vi "Graph Buffer.vi"(4 "Channel Names":string[](array[string]), 5 "Channels":T2, 6 "Data":sgl[](array[numeric]) format="%.2f", 7 "X Range":T3) -> (0 "LastValues":T1, 1 "Graph 2":sgl[][](array[numeric]) format="%.2f", 3 "Graph 1":sgl[][](array[numeric]) format="%.2f")   [LabVIEW 2015]
doc: "This VI acts as a buffer for the Housekeeping data, maintaining a record of the last 120 minutes of data and putting out the requested graphs.\n\nHK Buffer.vi by David Thomson Original Code Consulting\n September 2002 www.originalcode.com"
uses:
  X Range.ctl
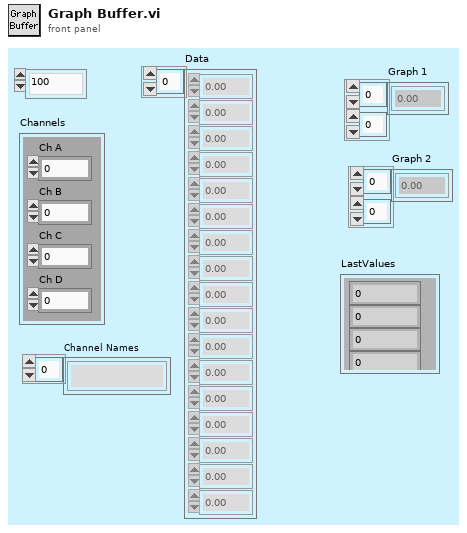
[diagram p1: front panel]
types:
  T1 = cluster{"Ch0":sgl, "Ch1":sgl, "Ch2":sgl, "Ch3":sgl}
  T2 = cluster{"Ch A":i32, "Ch B":i32, "Ch C":i32, "Ch D":i32}
  T3 = typedef "X Range.ctl" = enum16{"100", "300", "500", "1000", "3000", "5000", "10000", "20000", "30000", "40000", "60000"}
  T4 = cluster{"RT Channel":sgl, "RT Channel":sgl, "RT Channel":sgl, "RT Channel":sgl}
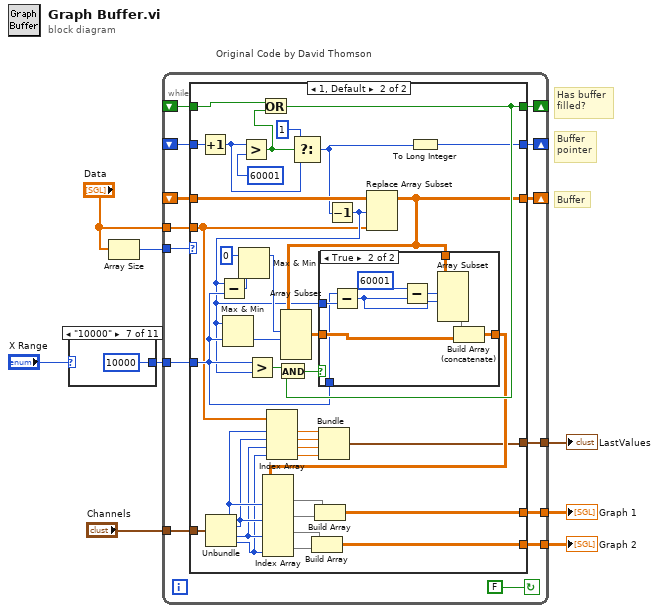
[diagram p0: block diagram]
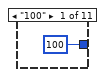
[diagram p2: hidden frame]
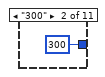
[diagram p3: hidden frame]
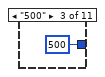
[diagram p4: hidden frame]
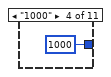
[diagram p5: hidden frame]
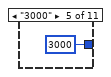
[diagram p6: hidden frame]
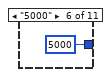
[diagram p7: hidden frame]
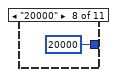
[diagram p8: hidden frame]
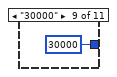
[diagram p9: hidden frame]
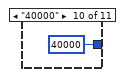
[diagram p10: hidden frame]
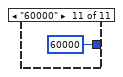
[diagram p11: hidden frame]
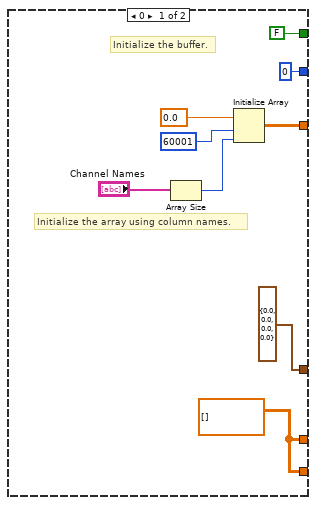
[diagram p12: hidden frame]
diagram:
  # "Buffer"
  # "Buffer\npointer"
  # "Has buffer\nfilled?"
  n1 = case shown="\"10000\"" "X Range" {
    tunnel: [100 ("y") 300 ("y") 500 ("y") 1000 ("y") 3000 ("y") 5000 ("y") 10000 ("y") 20000 ("y") 30000 ("y") 40000 ("y") 60000 ("y")] -> w5
    frame "100" {
    }
    frame "300" {
    }
    frame "500" {
    }
    frame "1000" {
    }
    frame "3000" {
    }
    frame "5000" {
    }
    frame "10000" {
    }
    frame "20000" {
    }
    frame "30000" {
    }
    frame "40000" {
    }
    frame "60000" {
    }
  }
  n2 = Array Size(array="Data") -> (size(s)=w8:i32)
  n3 = while "Original Code by David Thomson" {
    shift-right: [w31] -> _
    shift-left: _ -> [w29]
    shift-right: [w30] -> _
    shift-left: _ -> [w28]
    tunnel: w8 -> [w32]
    tunnel: "Data" -> [w27]
    tunnel: w5 -> [w26]
    shift-right: [w25] -> _
    shift-left: _ -> [w24]
    tunnel: "Channels" -> [w23]
    tunnel: [w22] -> w3
    tunnel: [w21] -> w2
    tunnel: [w20] -> w1
    stop <- FALSE continue-if-true
    n4 = case shown="1, Default" w32 {
      tunnel: [0 w65] -> w31
      tunnel: [w40 w71] -> w30
      tunnel: w29 -> [_ w67]
      tunnel: w28 -> [_ w78]
      tunnel: w27 -> [_ w53]
      tunnel: w26 -> [_ w59]
      tunnel: [FALSE w74] -> w25
      tunnel: w24 -> [_ w77]
      tunnel: w23 -> [_ w76]
      tunnel: [w37 w69] -> w22
      tunnel: [w37 w68] -> w21
      tunnel: [cluster{sgl, sgl, sgl, sgl} {0.0, 0.0, 0.0, 0.0} w44] -> w20
      frame 0 {
        w37 = sgl[][] []
        # "Initialize the array using column names."
        # "Initialize the buffer."
        n5 = Array Size(array="Channel Names") -> (size(s)=w35:i32)
        n6 = Initialize Array(sgl 0.0, 60001 ("dimension size"), w35) -> (w40:sgl[][])
      }
      frame 1, Default {
        n7 = Increment(x=w67) -> (x+1=w66:i32)
        n8 = Unbundle(w76) -> ("Ch A"=w52:i32, "Ch B"=w51:i32, "Ch C"=w50:i32, "Ch D"=w49:i32)
        n9 = Greater?(x=w66, y=60001) -> (0:w43:bool)
        n10 = Or(x=w77, y=w43) -> (x .or. y?=w74:bool)
        n11 = Index Array(array=w53, index #1=w52, index #2=w51, index #3=w50, index #4=w49) -> (element #1=w48:sgl, element #2=w47:sgl, element #3=w46:sgl, element #4=w45:sgl)
        n12 = Select(t=1 ("y"), s=w43, f=w66) -> (s? t:f=w60:i32)
        n13 = Bundle("RT Channel"=w48, "RT Channel"=w47, "RT Channel"=w46, "RT Channel"=w45) -> (w44:T4)  [unwired: 1 in]
        n14 = Decrement(x=w60) -> (x-1=w58:i32)
        n15 = Subtract(x=w58, y=w59) -> (x-y=w61:i32)
        n16 = Max & Min(x=w58, y=w59) -> (min(x,y)=w64:i32)  [unwired: 1 out]
        n17 = Max & Min(x=0 ("index"), y=w61) -> (max(x,y)=w62:i32)  [unwired: 1 out]
        n18 = Greater?(x=w59, y=w58) -> (0:w75:bool)
        n19 = And(x=w75, y=w74) -> (x .and. y?=w73:bool)
        n20 = Replace Array Subset(array=w78, new element=w53, index (row)=w58) -> (w71:sgl[][])  [unwired: 1 in]
        n21 = Array Subset(array=w71, index (row)=w62, length (row)=w64) -> (w72:sgl[][])  [unwired: 2 in]
        n22 = case shown="True" w73 {
          tunnel: [w81 w87] -> w70
          tunnel: w72 -> [w81 w88]
          tunnel: w71 -> [_ w90]
          tunnel: w58 -> [_ w84]
          tunnel: w59 -> [_ w82]
          frame False {
          }
          frame True {
            n23 = Subtract(x=w82, y=w84) -> (x-y=w83:i32)
            n24 = Subtract(x=60001 ("y"), y=w83) -> (x-y=w85:i32)
            n25 = Array Subset(array=w90, index (row)=w85, length (row)=w83) -> (w89:sgl[][])  [unwired: 2 in]
            n26 = Build Array (concatenate)(w89, w88) -> (w87:sgl[][])
          }
        }
        n27 = Index Array(array=w70, index (col) #1=w52, index (col) #2=w51, index (col) #3=w50, index (col) #4=w49) -> (element #1=w54:sgl[], element #2=w57:sgl[], element #3=w56:sgl[], element #4=w55:sgl[])  [unwired: 4 in]
        n28 = Build Array(w56, w55) -> (w68:sgl[][])
        n29 = Build Array(w54, w57) -> (w69:sgl[][])
        n30 = To Long Integer(number=w60) -> (32bit integer=w65:i32)
      }
    }
  }
  "Graph 1" <- w3
  "Graph 2" <- w2
  "LastValues" <- w1
